vi "AuMT8852B Status Byte Enable.vi"(5 "Flags in (all disabled)":T1 {"EUT Power State" items=["EUT power state disabled", "EUT power state enabled"]}, 7 "Set/Get (Set)":enum16{"Set", "Get"}(ring), 8 "error in (no error)":errorcluster, 10 "Value (-1)":i32=-1, 11 "VISA session":refnum<visa-resource-name>) -> (0 "error out":errorcluster, 2 "error code":i32, 3 "VISA session out":refnum<visa-resource-name>, 4 "Flags out":T1 {"EUT Power State" items=["EUT power state disabled", "EUT power state enabled"]}, 6 "Value out":i32)   [LabVIEW 2017]
doc: "Anritsu MT8852B Bluetooth Tester\n\nIndicates which bits of the IEE-488.2 standard Status Byte will cause a Service Request (SRQ). The value can be written as an integer (0-255), or as a cluster of flags.\n\nBit 5 - Message available - this bit is always set when there is data available to be read out of the output buffer and cleared when the output buffer is empty.\n\nBit 4 - Event status bit - this bit is set when a bit is set in the event register and the corresponding bit has been set in the event status enable register (ESE).\n\nBit 3 - Change bit - indicates that some change has occurred and the appropriate bit has been set in the CHG register.\n\nBit 2 - EUT Power State - This bit is set when the EUT is at either max or min power\n\nBit 1 - Equipment test fail - this bit is set when one of the equipment under test fail register bits has been set and the corresponding bit in the equipment under test fail register enable (ETE) bit has been set.\n\nBit 0 (least significant bit) - Instrument status - this bit is set when one of the instrument status bits has been set and the corresponding bit in the instrument status enable (INE) register has been set.\n\nINPUTS\nSet/Get - whether the values are being written to or read from the instrument.\nFlags - individual values to assign to the register.\nValue - integer value (0-255) to be written to the register. Leave this input unwired if you are using the Flags input.\n\nOUTPUTS\nFlags out - value of each bit in the register.\nValue out - integer value (0-255) of the register."
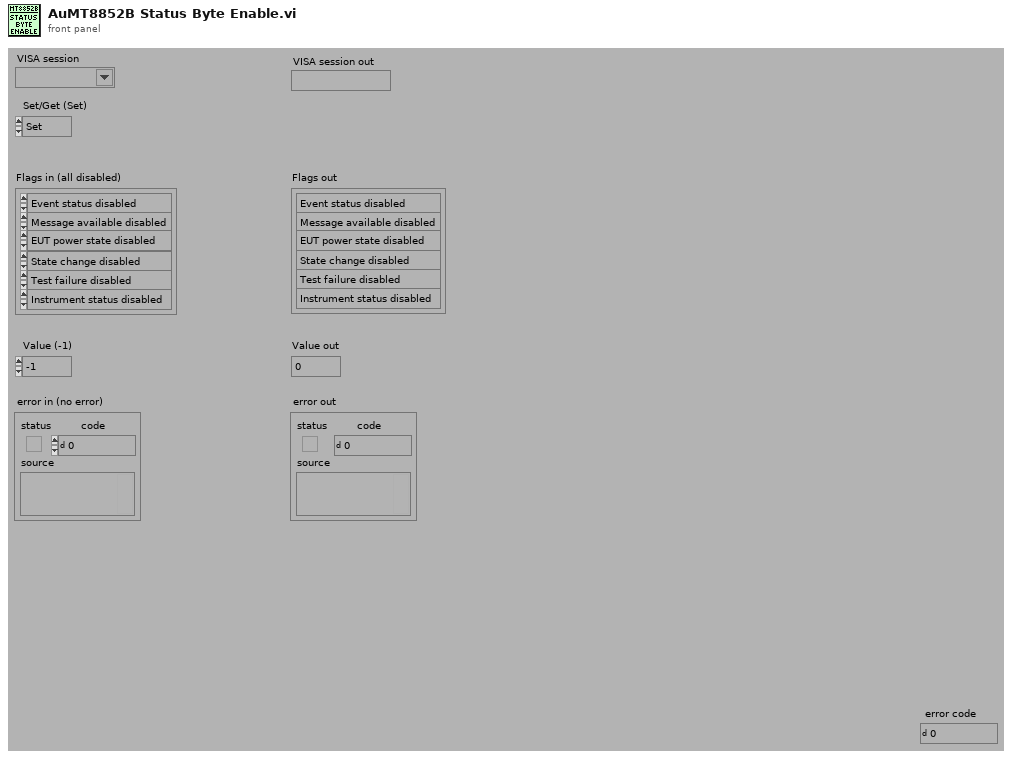
[diagram p1: front panel]
types:
  T1 = cluster{"Event status":enum16{"Event status disabled", "Event status enabled"}, "Message":enum16{"Message available disabled", "Message available enabled"}, "EUT Power State":u16, "State change":enum16{"State change disabled", "State change enabled"}, "Test failure":enum16{"Test failure disabled", "Test failure enabled"}, "Instrument status":enum16{"Instrument status disabled", "Instrument status enabled"}}
  T2 = enum16{"Simulate", "Range check", "Cache", "Query instrument status"}
  T3 = cluster{"[0]":i16, "[1]":i16, "[2]":i16, "[3]":i16, "[4]":i16, "[5]":i16, "[6]":i16, "[7]":i16}
  T4 = enum16{"Instrument status disabled", "Instrument status enabled"}
  T5 = enum16{"Test failure disabled", "Test failure enabled"}
  T6 = enum16{"State change disabled", "State change enabled"}
  T7 = enum16{"Message available disabled", "Message available enabled"}
  T8 = enum16{"Event status disabled", "Event status enabled"}
  T9 = cluster{bool, bool, bool, bool, bool, bool, bool, bool}
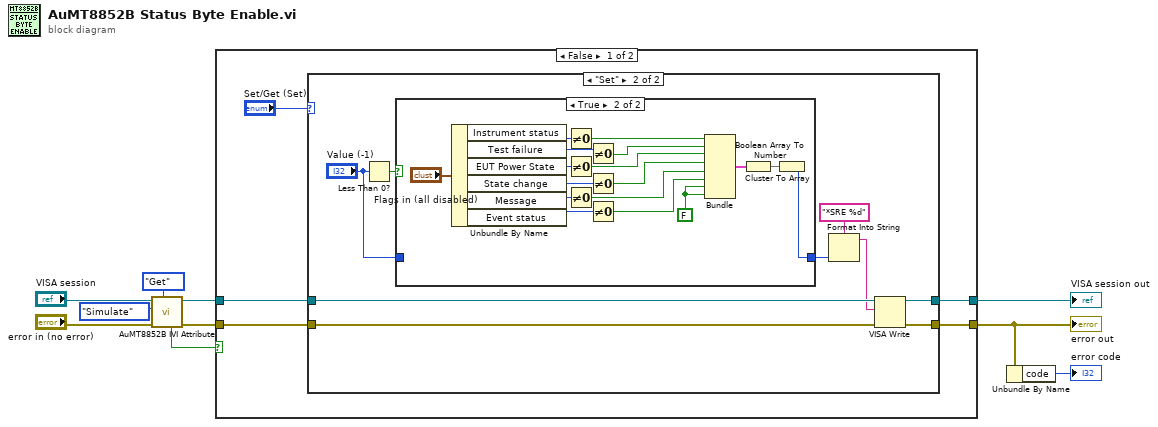
[diagram p0: block diagram]
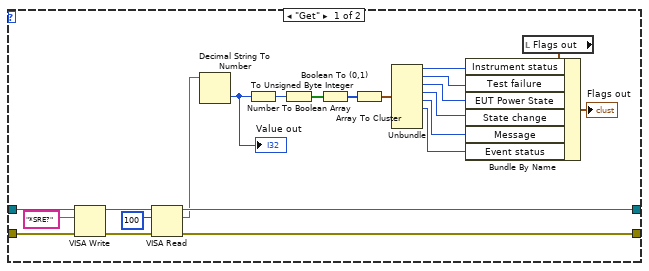
[diagram p2: hidden frame]
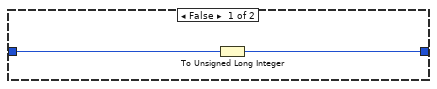
[diagram p3: hidden frame]
diagram:
  n1 = call <instrlib>:"AuMT8852B IVI Attribute.vi"("Set/Get (Set)"=enum16{"Set", "Get"}."Get", "error in (no error)"="error in (no error)", "Flag (Simulate)"=T2."Simulate", "VISA session"="VISA session") -> ("error out"=w6:errorcluster, "VISA session out"=w7:refnum<visa-resource-name>, "Value out"=w3:bool)  [unwired: 5 in]
  n2 = case shown="False" w3 {
    tunnel: [w12 w66] -> w1
    tunnel: [w13 w67] -> w8
    tunnel: w7 -> [w15 w67]
    tunnel: w6 -> [w14 w66]
    frame False {
      n3 = case shown="\"Set\"" "Set/Get (Set)" {
        tunnel: w15 -> [w37 w46]
        tunnel: w14 -> [w36 w45]
        tunnel: [w32 w42] -> w13
        tunnel: [w31 w41] -> w12
        frame "Get" {
          n4 = VISA Write(VISA resource name=w37, write buffer="*SRE?" ("write buffer (\"\")"), error in (no error)=w36) -> (VISA resource name out=w34:refnum<visa-resource-name>, error out=w33:errorcluster)  [unwired: 1 out]
          n5 = VISA Read(VISA resource name=w34, byte count=u32 100 ("byte count (0)"), error in (no error)=w33) -> (VISA resource name out=w32:refnum<visa-resource-name>, read buffer=w29:string, error out=w31:errorcluster)  [unwired: 1 out]
          n6 = Decimal String To Number(string=w29) -> (number=w23:i32)  [unwired: 2 in, 1 out]
          "Value out" <- w23
          n7 = To Unsigned Byte Integer(number=w23) -> (unsigned 8bit integer=w24:u8)
          n8 = Number To Boolean Array(number=w24) -> (Boolean array=w25:bool[])
          n9 = Boolean To (0,1)(Boolean=w25) -> (0, 1=w26:i16[])
          n10 = Array To Cluster(array=w26) -> (cluster=w27:T3)
          n11 = Unbundle(w27) -> ("[0]"=w22:i16, "[1]"=w21:i16, "[2]"=w17:i16, "[3]"=w16:i16, "[4]"=w20:i16, "[5]"=w19:i16)  [unwired: 2 out]
          n12 = local read "Flags out"() -> (w28:T1)
          n13 = Bundle By Name(cluster=w28, "Instrument status"=w22, "Test failure"=w21, "EUT Power State"=w17, "State change"=w16, "Message"=w20, "Event status"=w19) -> (→"Flags out":T1)
        }
        frame "Set" {
          n14 = Less Than 0?(x="Value (-1)") -> (x < 0?=w39:bool)
          n15 = case shown="True" w39 {
            tunnel: [w47 w62] -> w43
            tunnel: "Value (-1)" -> [w48 _]
            frame False {
              n16 = To Unsigned Long Integer(number=w48) -> (unsigned 32bit integer=w47:u32)
            }
            frame True {
              w51 = FALSE
              n17 = Unbundle By Name("Flags in (all disabled)") -> ("Instrument status"=w65:T4, "Test failure"=w61:T5, "EUT Power State"=w60:u16, "State change"=w50:T6, "Message"=w59:T7, "Event status"=w58:T8)
              n18 = Not Equal To 0?(x=w65) -> (x != 0?=w56:bool)
              n19 = Not Equal To 0?(x=w60) -> (x != 0?=w54:bool)
              n20 = Not Equal To 0?(x=w59) -> (x != 0?=w53:bool)
              n21 = Not Equal To 0?(x=w61) -> (x != 0?=w55:bool)
              n22 = Not Equal To 0?(x=w50) -> (x != 0?=w49:bool)
              n23 = Not Equal To 0?(x=w58) -> (x != 0?=w52:bool)
              n24 = Bundle(w56, w55, w54, w49, w53, w52, w51, w51) -> (w64:T9)  [unwired: 1 in]
              n25 = Cluster To Array(cluster=w64) -> (array=w63:bool[])
              n26 = Boolean Array To Number(Boolean array=w63) -> (number=w62:u32)
            }
          }
          n27 = Format Into String(format string="*SRE %d" ("Format String"), w43) -> (resulting string=w40:string)  [unwired: 2 in, 1 out]
          n28 = VISA Write(VISA resource name=w46, write buffer=w40, error in (no error)=w45) -> (VISA resource name out=w42:refnum<visa-resource-name>, error out=w41:errorcluster)  [unwired: 1 out]
        }
      }
    }
    frame True {
    }
  }
  "error out" <- w1
  "VISA session out" <- w8
  n29 = Unbundle By Name(w1) -> ("code"=→"error code":i32)
